vi "Combine Disp Offsets.vi"(8 "error in (no error)":errorcluster) -> (0 "error out":errorcluster)   [LabVIEW 2009]
uses:
  Global Data/Transactions/Dataset Type.ctl
  Global Data/Transactions/Dataset Source.ctl
  Global Data/Transactions/Dataset Transaction Id.ctl
  Apps/Yes No Button.ctl
  Data Access Objects/Metadata/DAO Actions.ctl
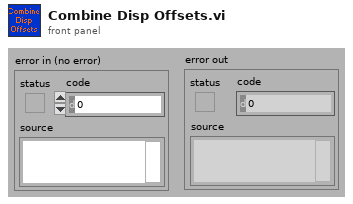
[diagram p1: front panel]
types:
  T1 = typedef "Dataset Transaction Id.ctl" = cluster{"Dataset Source":T2, "Dataset Type":T3, "Hold":T4, "Volts":T4, "Tag":string}
  T2 = typedef "Dataset Source.ctl" = enum16{"LBCB 1", "LBCB 2", "Combined", "External Sensors"}
  T3 = typedef "Dataset Type.ctl" = enum16{"LVDT", "Load Cell", "Actuator Command", "Servo Error", "Displacement Command", "Displacement", "Force"}
  T4 = typedef "Yes No Button.ctl" = bool
  T5 = typedef "DAO Actions.ctl" = enum16{"Init", "Get", "Set"}
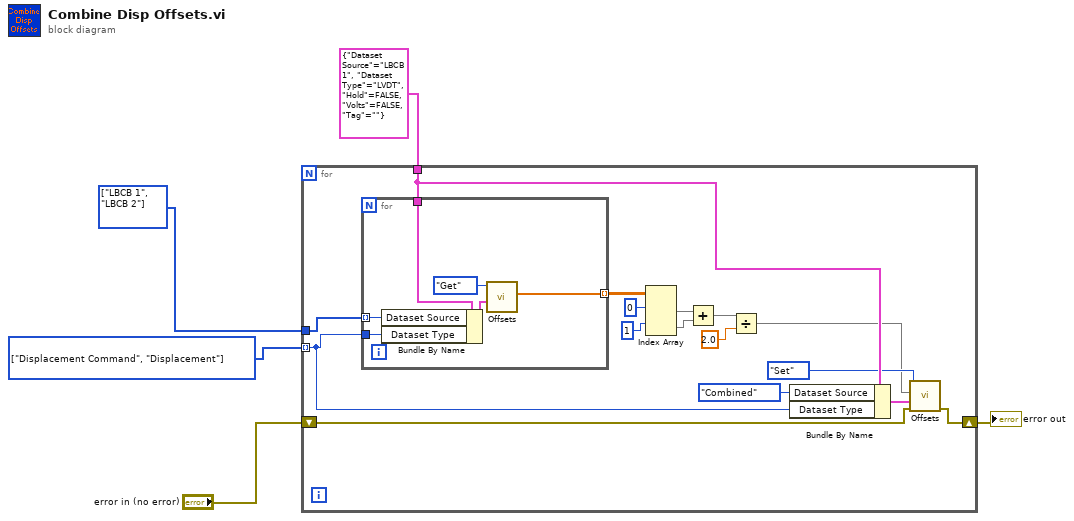
[diagram p0: block diagram]
diagram:
  w4 = T2[] [enum."LBCB 1", enum."LBCB 2"] items=["LBCB 1", "LBCB 2", "Combined", "External Sensors"]
  w3 = T3[] [enum."Displacement Command", enum."Displacement"] items=["LVDT", "Load Cell", "Actuator Command", "Servo Error", "Displacement Command", "Displacement", "Force"]
  n1 = for {
    tunnel: T1 {"Dataset Source"=enum."LBCB 1", "Dataset Type"=enum."LVDT", "Hold"=FALSE, "Volts"=FALSE, "Tag"=""} ("Dataset Trans Id") -> [w20]
    tunnel: w4 -> [w21]
    tunnel: w3 -> [w18] mode=indexing
    shift-right: [w6] -> w1
    shift-left: "error in (no error)" -> [w7]
    n2 = for {
      tunnel: w20 -> [w26]
      tunnel: w21 -> [w24] mode=indexing
      tunnel: w18 -> [w23]
      tunnel: [w22] -> w19 mode=indexing
      n3 = Bundle By Name(cluster=w26, "Dataset Source"=w24, "Dataset Type"=w23) -> (w25:T1)
      n4 = call "Offsets.vi"("Dataset Trans Id"=w25, "DAO Actions"=DAO_Actions."Get") -> ("Data Out"=w22:dbl[])  [unwired: 7 in, 2 out]
    }
    n5 = Index Array(array=w19, index (row) #1=0 ("index (row)"), index (row) #2=1 ("index (row)")) -> (element #1=w15:dbl[], element #2=w14:dbl[])  [unwired: 2 in]
    n6 = Add(x=w15, y=w14) -> (x+y=w13:dbl[])
    n7 = Divide(x=w13, y=2.0) -> (x/y=w9:dbl[])
    n8 = Bundle By Name(cluster=w20, "Dataset Source"=Dataset_Source."Combined", "Dataset Type"=w18) -> (w12:T1)
    n9 = call "Offsets.vi"("error in (no error)"=w7, "Dataset Trans Id"=w12, "Data In"=w9, "DAO Actions"=DAO_Actions."Set") -> ("error out"=w6:errorcluster)  [unwired: 5 in, 2 out]
  }
  "error out" <- w1
